vi "Get Position Piezo.vi"(5 "Piezo State":T2, 7 "Counter Time":i32, 8 "error in (no error)":errorcluster, 9 "notifier out":refnum<notifier>, 11 "Cluster 3":T1={"serial number"="Dev5/ao0", "handle"=10, "status"=0, "range"=0}) -> (0 "error out":errorcluster)   [LabVIEW 2013, in "Piezo.lvlib"]
uses:
  Piezo/Piezo.lvlib
  Piezo/Piezo State.ctl
  Piezo/Piezo display.ctl
  Hardware Configuration Piezo NEW.ctl
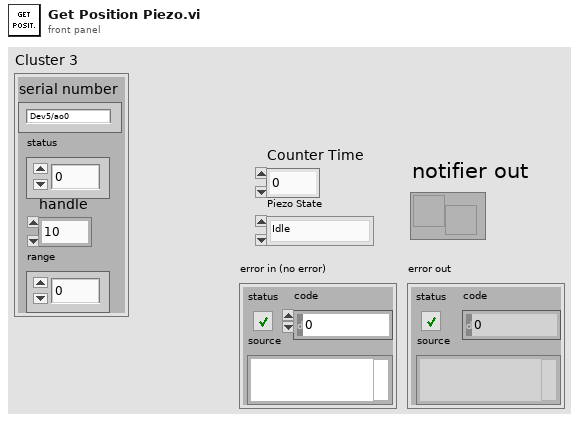
[diagram p1: front panel]
types:
  T1 = typedef "Hardware Configuration Piezo NEW.ctl" = cluster{"serial number":string, "handle":i32, "status":i32, "range":i32}
  T2 = typedef "Piezo.lvlib/Piezo State.ctl" = enum16{"Idle", "Acquiring"}
  T3 = typedef "Piezo.lvlib/Piezo display.ctl" = cluster{"PiezoPosition":sgl, "Counter Time":i32}
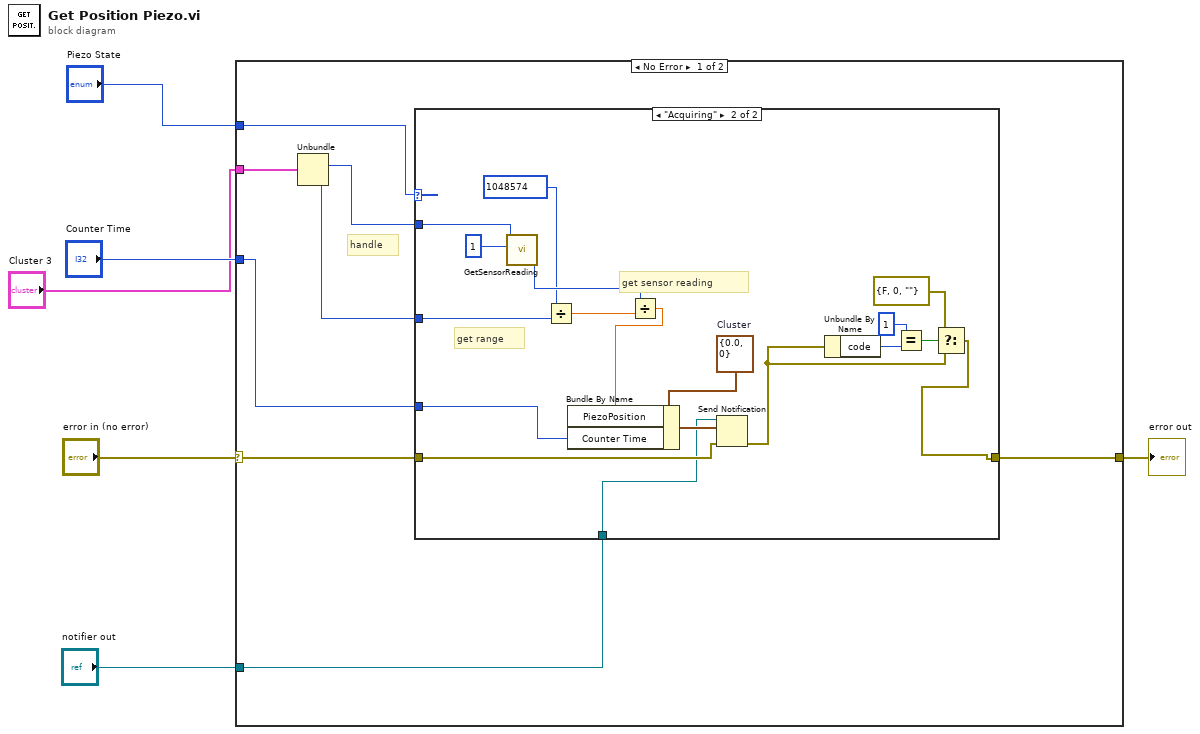
[diagram p0: block diagram]
diagram:
  n1 = case shown="No Error" "error in (no error)" {
    selector: "error in (no error)" -> [w13 w34]
    tunnel: [w12 w34] -> w5
    tunnel: "Piezo State" -> [w8 _]
    tunnel: "Counter Time" -> [w14 _]
    tunnel: "notifier out" -> [w11 _]
    tunnel: "Cluster 3" -> [w10 _]
    frame No Error {
      # "handle"
      n2 = Unbundle(w10) -> ("handle"=w9:i32, "range"=w7:i32)  [unwired: 2 out]
      n3 = case shown="\"Acquiring\"" w8 {
        tunnel: w14 -> [_ w31]
        tunnel: w11 -> [_ w25]
        tunnel: w13 -> [w15 w32]
        tunnel: [w15 w23] -> w12
        tunnel: w9 -> [_ w22]
        tunnel: w7 -> [_ w16]
        frame "Idle", Default {
        }
        frame "Acquiring" {
          w30 = T3 {"PiezoPosition"=0.0, "Counter Time"=0}  # Cluster
          # "get sensor reading"
          # "get range"
          n4 = call "GetSensorReading.vi"("Handle"=w22, "Controller Channel"=1) -> ("Sensor Reading"=w20:i32)  [unwired: 7 in, 1 out]
          n5 = Divide(x=1048574, y=w16) -> (x/y=w19:dbl)
          n6 = Divide(x=w20, y=w19) -> (x/y=w17:dbl)
          n7 = Bundle By Name(cluster=w30, "PiezoPosition"=w17, "Counter Time"=w31) -> (w33:T3)
          n8 = Send Notification(notification=w33, notifier=w25, error in (no error)=w32) -> (error out=w24:errorcluster)  [unwired: 1 out]
          n9 = Unbundle By Name(w24) -> ("code"=w29:i32)
          n10 = Equal?(x=1, y=w29) -> (x = y?=w27:bool)
          n11 = Select(t=errorcluster {"status"=FALSE, "code"=0, "source"=""} ("error constant"), s=w27, f=w24) -> (s? t:f=w23:errorcluster)
        }
      }
    }
    frame Error {
    }
  }
  "error out" <- w5
